vi "gRPC_ATS.vi"(11 "CommandLineIn":string[](array[string])) -> (2 "source":string, 3 "return code":i32)   [LabVIEW 2019]
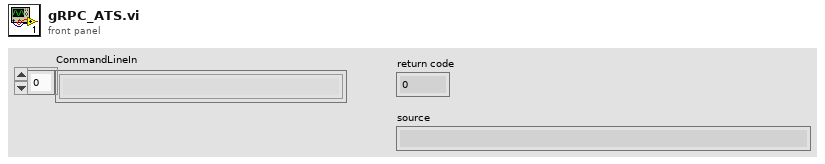
[diagram p1: front panel]
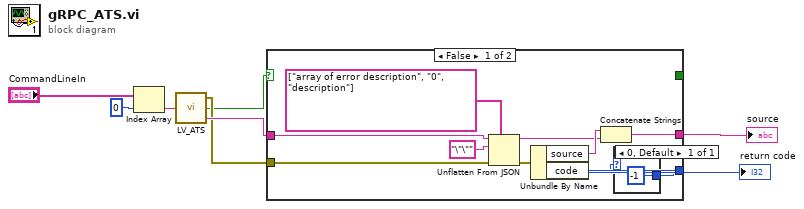
[diagram p0: block diagram]
diagram:
  n1 = Index Array(array="CommandLineIn", index=0) -> (element=w7:string)
  n2 = call "LV_ATS.vi"("test json in"=w7) -> ("formatted test json out"=w3:string, "PASS"=w1:bool, "error out"=w2:errorcluster)  [unwired: 1 in, 1 out]
  n3 = case shown="False" w1 {
    selector: w1 -> [_ w20]
    tunnel: [_ w20] -> _
    tunnel: w3 -> [w18 _]
    tunnel: w2 -> [w13 _]
    tunnel: [w11 _] -> w4
    tunnel: [w9 _] -> w5
    frame False {
      n4 = Unflatten From JSON(path=string[] ["array of error description", "0", "description"], JSON string=w18, type and defaults="\"\"", error in (no error)=w13) -> (value=w15:string, error out=w12:errorcluster)  [unwired: 3 in]
      n5 = Unbundle By Name(w12) -> ("source"=w17:string, "code"=w10:i32)
      n6 = Concatenate Strings(w17, w15) -> (w11:string)
      n7 = case shown="0, Default" w10 {
        tunnel: [-1] -> w9
        frame 0, Default {
        }
      }
    }
    frame True {
    }
  }
  "return code" <- w5
  "source" <- w4
